vi "Convert Timestamp to String.vi"(11 "Calibration Info":T1) -> (3 "String":string)   [LabVIEW 2017]
doc: "Takes \"Next Cal Date\" from <B>Calibration Info</B> and turns it into a string to be displayed."
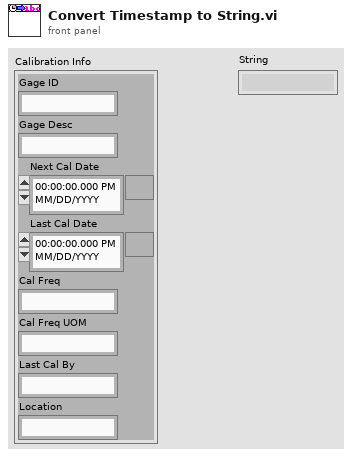
[diagram p1: front panel]
types:
  T1 = cluster{"Gage ID":string, "Gage Desc":string, "Next Cal Date":timestamp, "Last Cal Date":timestamp, "Cal Freq":string, "Cal Freq UOM":string, "Last Cal By":string, "Location":string}
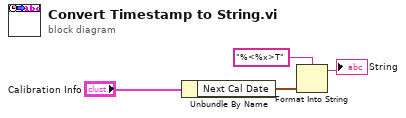
[diagram p0: block diagram]
diagram:
  n1 = Unbundle By Name("Calibration Info") -> ("Next Cal Date"=w1:timestamp)
  n2 = Format Into String(format string="%<%x>T", w1) -> (resulting string=→"String":string)  [unwired: 2 in, 1 out]
